vi "State_Machine.vi"(8 "error in (no error)":errorcluster caption="entrée d'erreur (pas d'erreur)", 11 "Delay en entrée":refnum<class "P2056_ExtractLog.lvclass">) -> (0 "error out":errorcluster caption="sortie d'erreur", 2 "Json_String":string, 3 "Delay en sortie":refnum<class "P2056_ExtractLog.lvclass">)   [LabVIEW 2020, in "Library Test.lvlib" / "P2056_ExtractLog.lvclass"]
uses:
  P2056_ExtractLog.lvclass
  C:/Users/ngarcin/OneDrive - Altyor/Standard TB/Suite TB45/Class/Test/Test (Default)/Test (Default).lvclass
  Commun VI/TypeDef/Variable Printable.ctl
  Read CSV File/CSV_File (Default)/Class CSV_File.lvclass
  C:/Users/ngarcin/OneDrive - Altyor/Standard TB/Suite TB45/Class/Read CSV File/Class File (Default)/Class File (Default).lvclass
  JSON API/JSON Value/Set from JSON string.vi
  JSON API/JSON Value/JSON Value.lvclass
  Commun VI/Library Commun.lvlib
  JSON API/Variant JSON/Variant JSON.lvlib
  JSON API/Get Polymorphic/JSON GetSet.lvlib
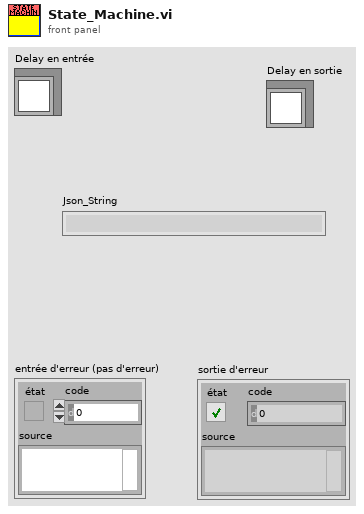
[diagram p1: front panel]
types:
  T1 = typedef "Variable Printable.ctl" = string
  T2 = enum16{"Get Variable", "Get All Variables", "Set Variable", "Delete Variable", "Delete All Variable"}
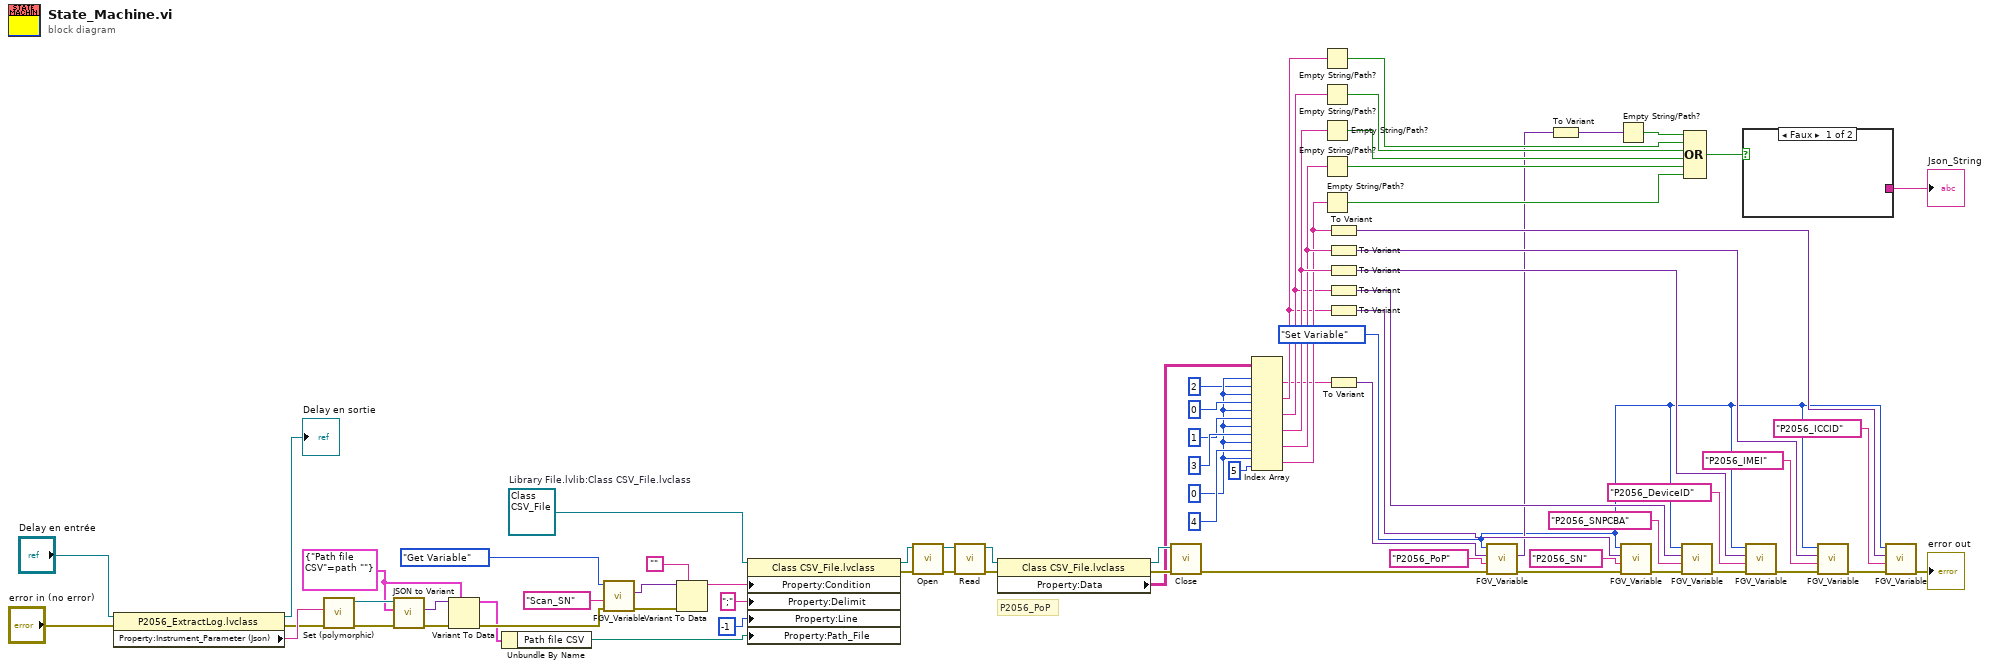
[diagram p0: block diagram]
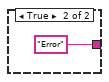
[diagram p2: hidden frame]
diagram:
  w11 = 0 ("indice (ligne)")
  w49 = cluster{"Path file CSV":path} {"Path file CSV"=path ""}
  w60 = refnum<class "Class CSV_File.lvclass"> refnum  # Library File.lvlib:Class CSV_File.lvclass
  w1 = T2."Set Variable" ("Function")
  # "P2056_PoP"
  n1 = property class="P2056_ExtractLog.lvclass"(reference="Delay en entrée", error in="error in (no error)") -> (reference out=→"Delay en sortie":refnum<class "P2056_ExtractLog.lvclass">, error out=w50:errorcluster, "Property:Instrument_Parameter (Json)"=w51:string)
  n2 = call-poly "Set (polymorphic).vi"("error in (no error)"=w50, "JSON stream"=w51) -> ("error out"=w53:errorcluster, "JSON Value out"=w55:refnum<class "JSON Value.lvclass">)  [unwired: 7 in, 1 out]
  n3 = call "JSON to Variant.vi"("error in (no error)"=w53, "Variant (Data Type)"=w49, "JSON Value"=w55) -> ("error out"=w54:errorcluster, "Variant out"=w52:variant)  [unwired: 7 in]
  n4 = Variant To Data(error in=w54, type=w49, Variant=w52) -> (data=w44:cluster{"Path file CSV":path}, error out=w45:errorcluster)
  n5 = Unbundle By Name(w44) -> ("Path file CSV"=w59:path)
  n6 = call "FGV_Variable.vi"("error in (no error)"=w45, "Variable"=T1 "Scan_SN", "Function"=T2."Get Variable") -> ("error out"=w72:errorcluster, "Data Out"=w66:variant)  [unwired: 6 in, 1 out]
  n7 = Variant To Data(error in=w72, type="", Variant=w66) -> (data=w58:string)  [unwired: 1 out]
  n8 = property class="Class CSV_File.lvclass"(reference=w60, "Property:Condition"=w58, "Property:Delimit"=";" ("Delimit"), "Property:Line"=i16 -1 ("Line"), "Property:Path_File"=w59) -> (reference out=w63:refnum<class "Class CSV_File.lvclass">, error out=w62:errorcluster)  [unwired: 1 in]
  n9 = call-dynamic "Open.vi"("error in (no error)"=w62, "Class CSV_File (Default) en entrée"=w63) -> ("error out"=w65:errorcluster, "Class CSV_File (Default) en sortie"=w64:refnum<class "Class CSV_File.lvclass">)  [unwired: 8 in]
  n10 = call-dynamic "Read.vi"("error in (no error)"=w65, "Class CSV_File (Default) en entrée"=w64) -> ("error out"=w70:errorcluster, "Class CSV_File (Default) en sortie"=w68:refnum<class "Class CSV_File.lvclass">)  [unwired: 8 in]
  n11 = property class="Class CSV_File.lvclass"(reference=w68, error in=w70) -> (reference out=w67:refnum<class "Class CSV_File.lvclass">, error out=w69:errorcluster, "Property:Data"=w61:string[][])
  n12 = call-dynamic "Close.vi"("error in (no error)"=w69, "Class CSV_File (Default) en entrée"=w67) -> ("error out"=w4:errorcluster)  [unwired: 8 in, 1 out]
  n13 = Index Array(array=w61, index (row) #1=w11, index (col) #1=2 ("indice désactivé (col)"), index (row) #2=w11, index (col) #2=0 ("indice désactivé (col)"), index (row) #3=w11, index (col) #3=1 ("indice désactivé (col)"), index (row) #4=w11, index (col) #4=3 ("indice désactivé (col)"), index (row) #5=w11, index (col) #5=4 ("indice désactivé (col)"), index (row) #6=w11, index (col) #6=5 ("indice désactivé (col)")) -> (element #1=w2:string, element #2=w14:string, element #3=w20:string, element #4=w28:string, element #5=w27:string, element #6=w26:string)
  n14 = Empty String/Path?(string/path=w14) -> (empty?=w13:bool)
  n15 = Empty String/Path?(string/path=w20) -> (empty?=w22:bool)
  n16 = Empty String/Path?(string/path=w28) -> (empty?=w30:bool)
  n17 = Empty String/Path?(string/path=w27) -> (empty?=w31:bool)
  n18 = Empty String/Path?(string/path=w26) -> (empty?=w32:bool)
  n19 = To Variant(anything=w26) -> (Variant=w36:variant)
  n20 = To Variant(anything=w27) -> (Variant=w37:variant)
  n21 = To Variant(anything=w28) -> (Variant=w38:variant)
  n22 = To Variant(anything=w20) -> (Variant=w19:variant)
  n23 = To Variant(anything=w14) -> (Variant=w16:variant)
  n24 = To Variant(anything=w2) -> (Variant=w9:variant)
  n25 = call "FGV_Variable.vi"("error in (no error)"=w4, "Variable"=T1 "P2056_PoP", "Data In"=w9, "Function"=w1) -> ("error out"=w3:errorcluster, "Data Out"=w7:variant)  [unwired: 5 in, 1 out]
  n26 = To Variant(anything=w7) -> (Variant=w6:variant)
  n27 = Empty String/Path?(string/path=w6) -> (empty?=w5:bool)
  n28 = call "FGV_Variable.vi"("error in (no error)"=w3, "Variable"=T1 "P2056_SN", "Data In"=w16, "Function"=w1) -> ("error out"=w15:errorcluster)  [unwired: 5 in, 2 out]
  n29 = call "FGV_Variable.vi"("error in (no error)"=w15, "Variable"=T1 "P2056_SNPCBA", "Data In"=w19, "Function"=w1) -> ("error out"=w21:errorcluster)  [unwired: 5 in, 2 out]
  n30 = Compound Arithmetic op=OR ("Opérateur arithmétique")(w5, w13, w22, w30, w31, w32) -> (w25:bool)
  n31 = case shown="Faux" w25 {
    tunnel: [_ "Error"] -> w24
    frame False {
    }
    frame True {
    }
  }
  "Json_String" <- w24
  n32 = call "FGV_Variable.vi"("error in (no error)"=w21, "Variable"=T1 "P2056_DeviceID", "Data In"=w38, "Function"=w1) -> ("error out"=w40:errorcluster)  [unwired: 5 in, 2 out]
  n33 = call "FGV_Variable.vi"("error in (no error)"=w40, "Variable"=T1 "P2056_IMEI", "Data In"=w37, "Function"=w1) -> ("error out"=w39:errorcluster)  [unwired: 5 in, 2 out]
  n34 = call "FGV_Variable.vi"("error in (no error)"=w39, "Variable"=T1 "P2056_ICCID", "Data In"=w36, "Function"=w1) -> ("error out"=→"error out":errorcluster)  [unwired: 5 in, 2 out]
